vi "Schedule.EditFunction.vi"(8 "error in (no error)":errorcluster, 10 "Settings":string, 11 "ObjectSettings in":refnum<class "ObjectSettings.lvclass">) -> (0 "error out":errorcluster, 2 "Settings Out":string, 3 "ObjectSettings out":refnum<class "ObjectSettings.lvclass">)   [LabVIEW 2019, in "ObjectSettings.lvclass"]
uses:
  ObjectSettings.lvclass
  <vilib>/measure/NI_MABase.lvlib
  subVIs/typedefs/Schedule Types/Schedule--Function Generator.ctl
panel:
  out "Waveform Graph":dbl[](graph)
  in  "Signal Type":T1(ring) caption="Enum"
  in  "Duty Cycle (%)":dbl caption="Numeric"
  in  "Cycle Number":dbl caption="Numeric"
  in  "Max":dbl caption="Numeric"
  in  "Samples (Testing)":dbl caption="Numeric"
  in  "Min":dbl caption="Numeric"
  in  "Phase":dbl caption="Numeric"
  in  "Frequency":dbl caption="Numeric"
  in  "OK":bool
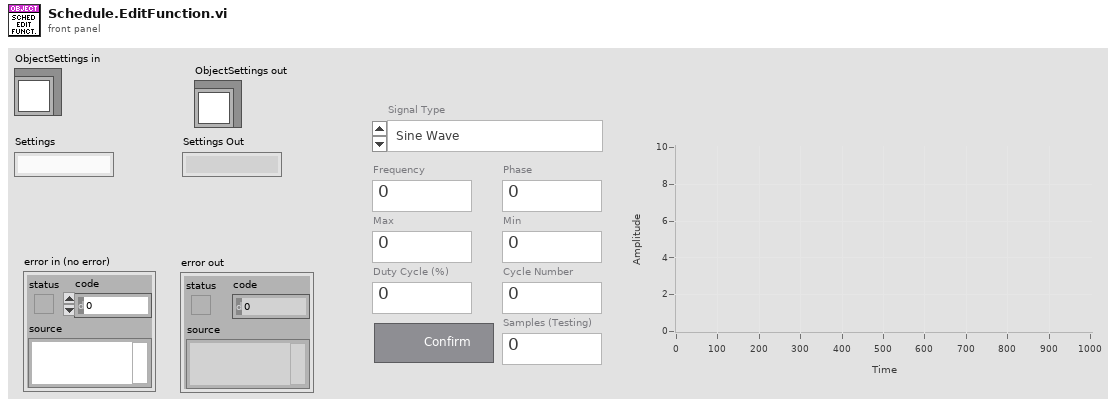
[diagram p1: front panel]
types:
  T1 = enum16{"Sine Wave", "Triangle Wave", "Square Wave", "Sawtooth Wave"}
  T2 = enum32{"Invalid", "Standard", "Closed", "Hidden", "Minimized", "Maximized"}
  T3 = enum32{"invalid app kind", "Development System", "Run Time System", "Student Edition", "Embedded LabVIEW", "Evaluation", "Custom"}
  T4 = typedef "Schedule--Function Generator.ctl" = cluster{"Min Value":dbl, "Max Value":dbl, "Duty Cycle (%)":dbl, "Signal Type":u16, "Cycle Number":dbl, "Phase (degrees)":dbl}
  T5 = cluster{"Core":cluster{"Current VI Reference":refnum<vi>, "Close Panel on Exit?":bool}, "ObjectSettings":refnum<class "ObjectSettings.lvclass">, "Settings":string, "Signal Type":enum16{"Sine Wave", "Triangle Wave", "Square Wave", "Sawtooth Wave"}, "Frequency":dbl, "Max":dbl, "Min":dbl, "Phase":dbl, "Samples (Testing)":dbl, "Cycle Number":dbl, "Duty Cycle (%)":dbl}
  T6 = cluster{"Current VI Reference":refnum<vi>, "Close Panel on Exit?":bool}
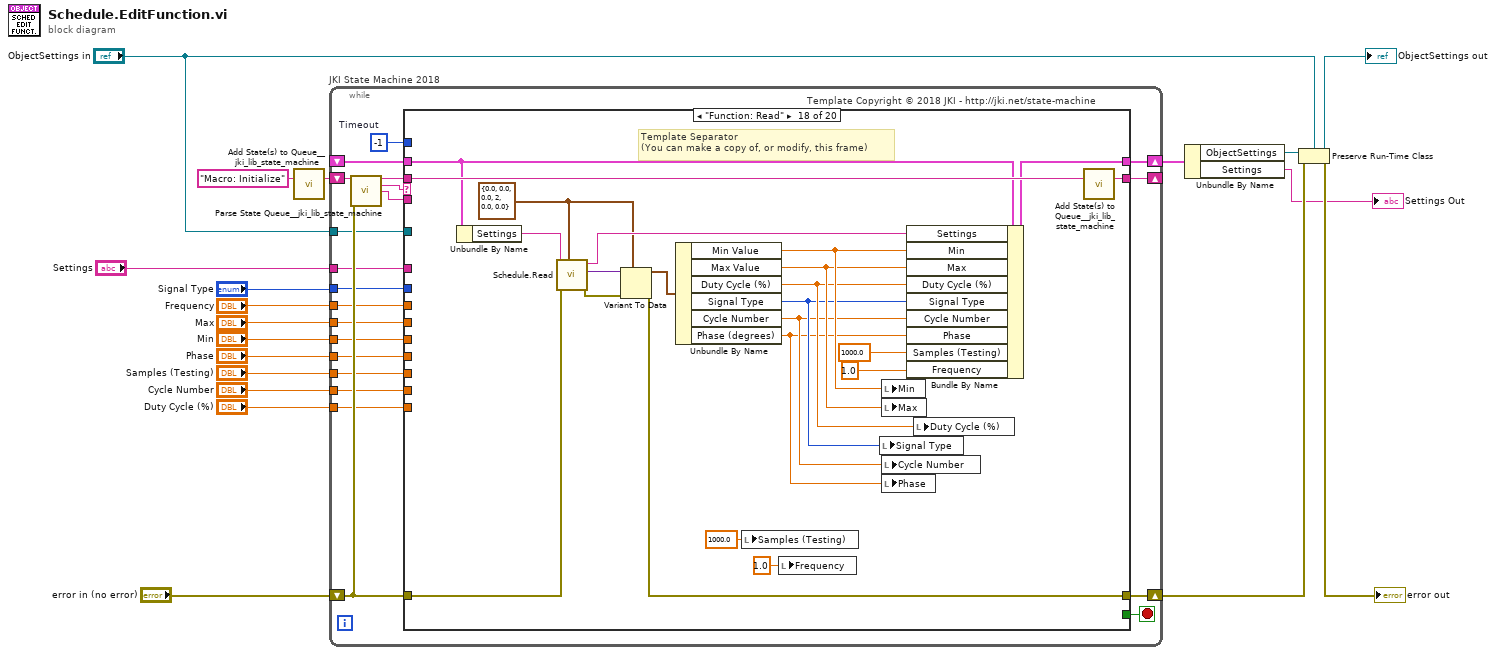
[diagram p0: block diagram]
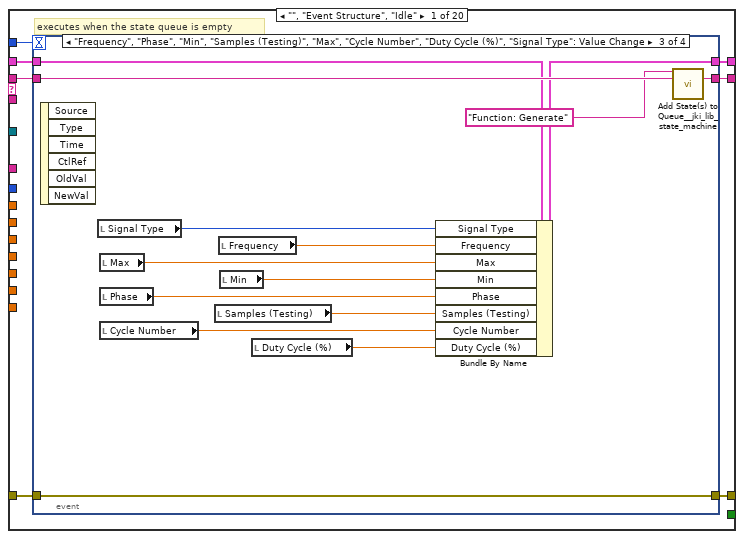
[diagram p2: hidden frame]
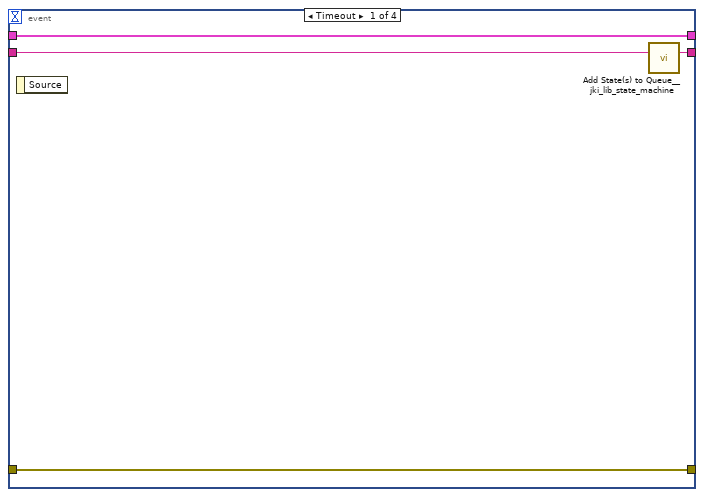
[diagram p3: hidden frame]
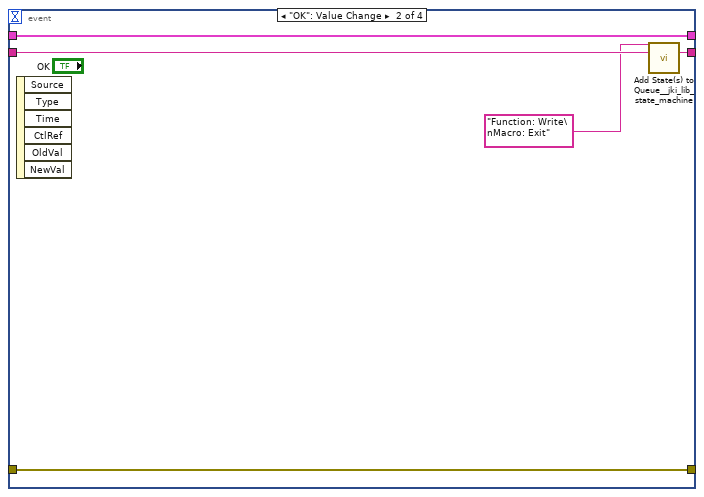
[diagram p4: hidden frame]
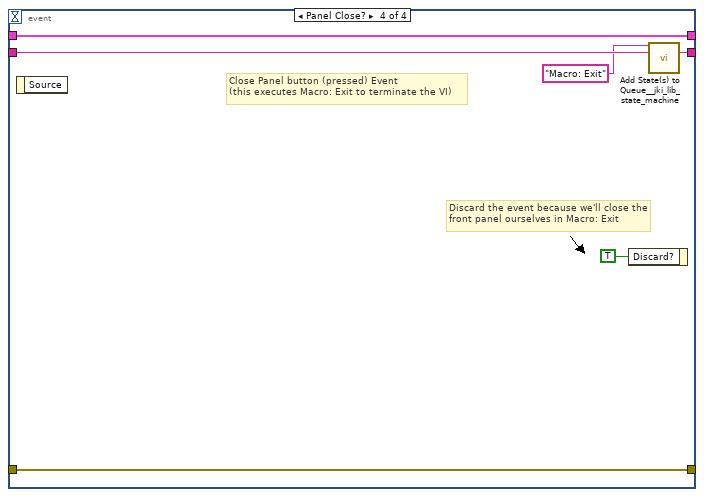
[diagram p5: hidden frame]
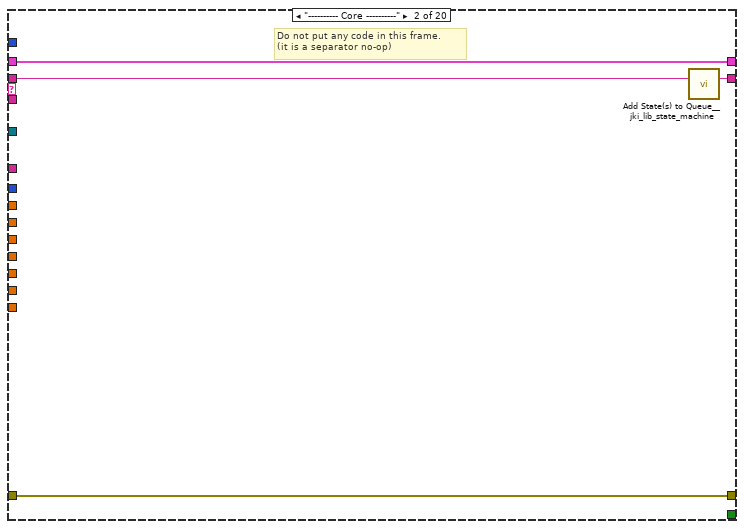
[diagram p6: hidden frame]
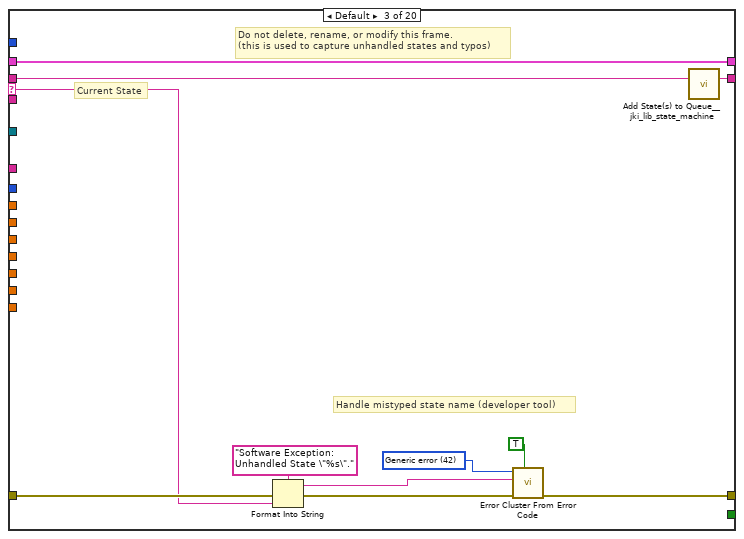
[diagram p7: hidden frame]
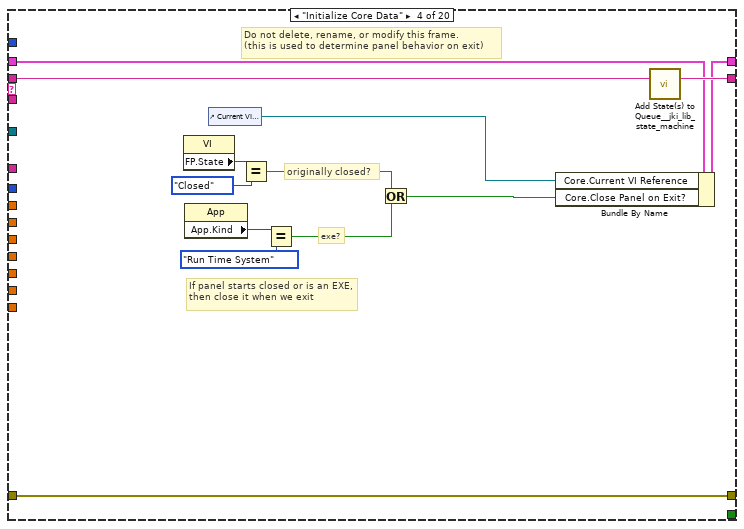
[diagram p8: hidden frame]
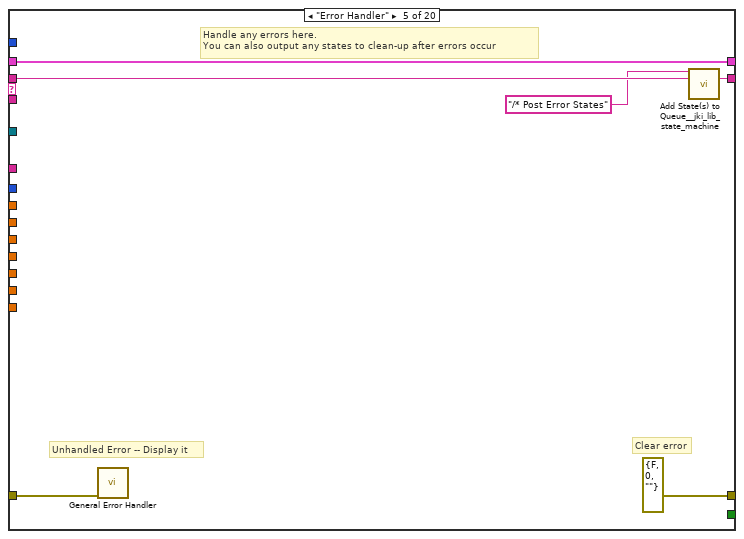
[diagram p9: hidden frame]
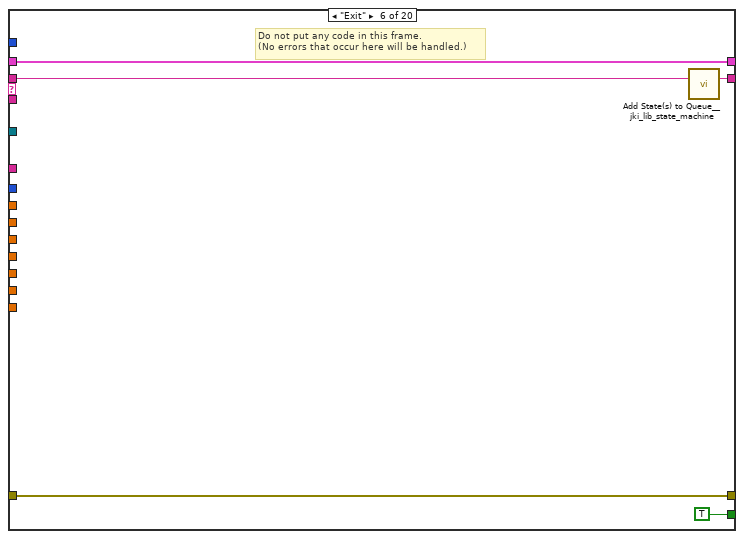
[diagram p10: hidden frame]
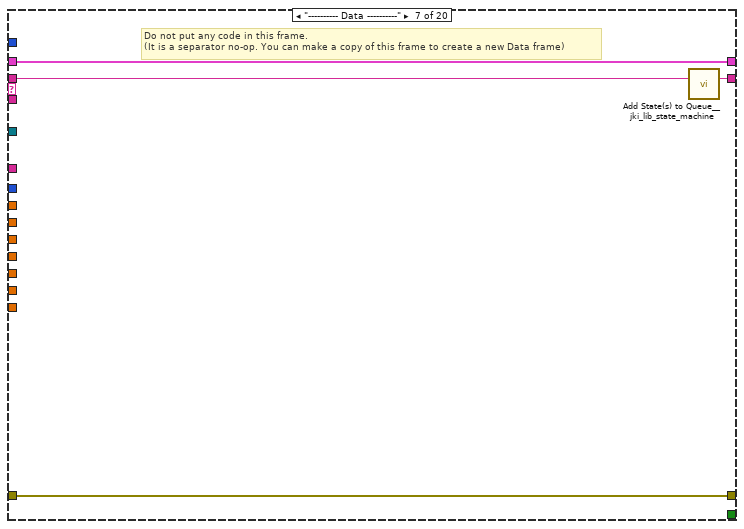
[diagram p11: hidden frame]
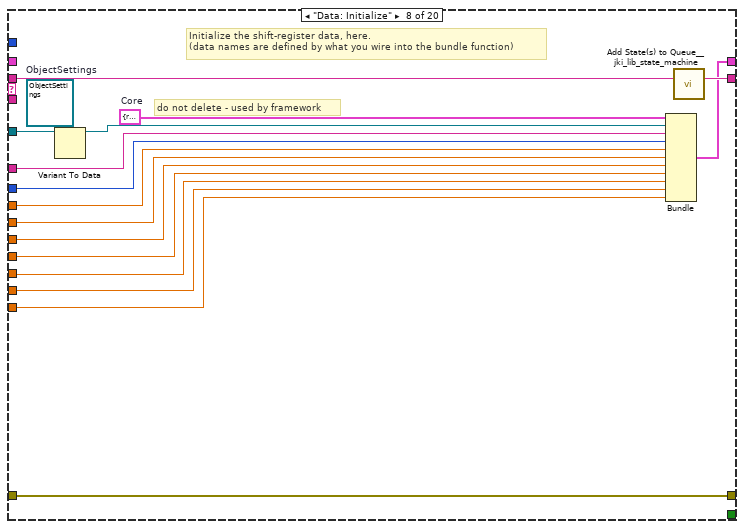
[diagram p12: hidden frame]
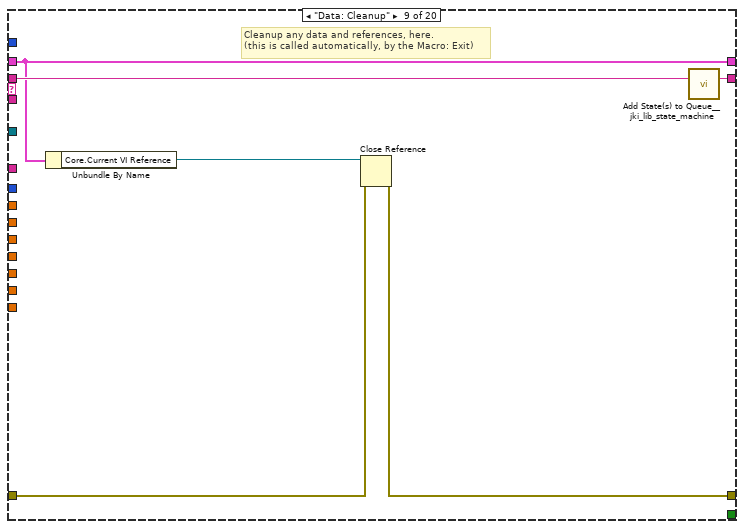
[diagram p13: hidden frame]
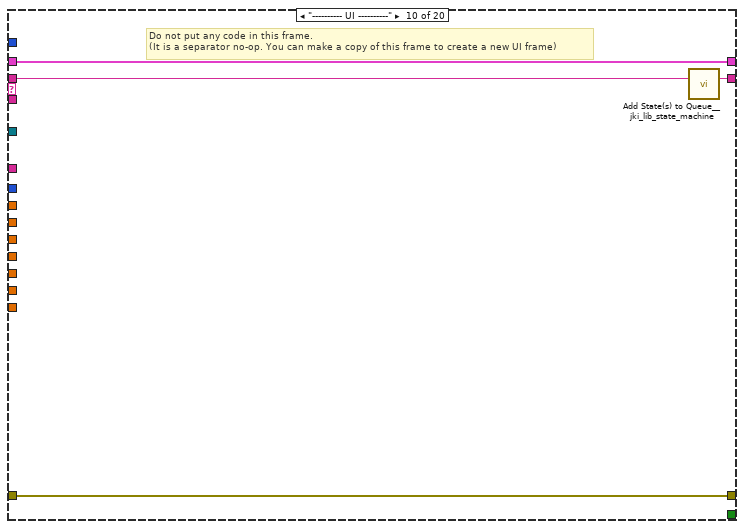
[diagram p14: hidden frame]
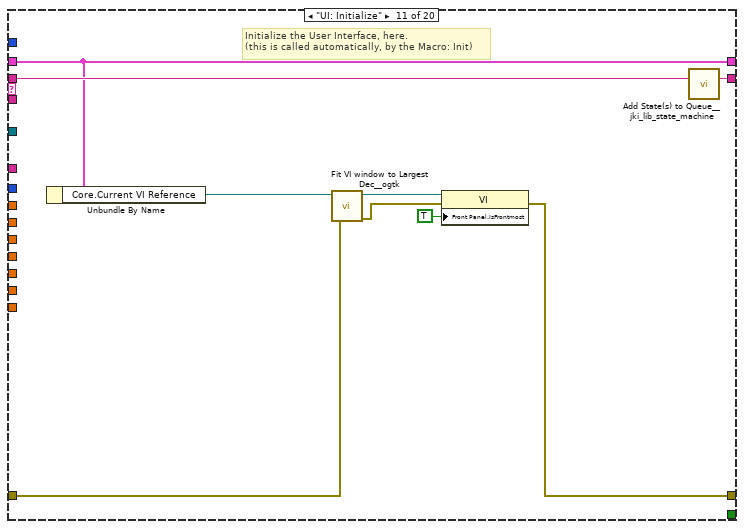
[diagram p15: hidden frame]
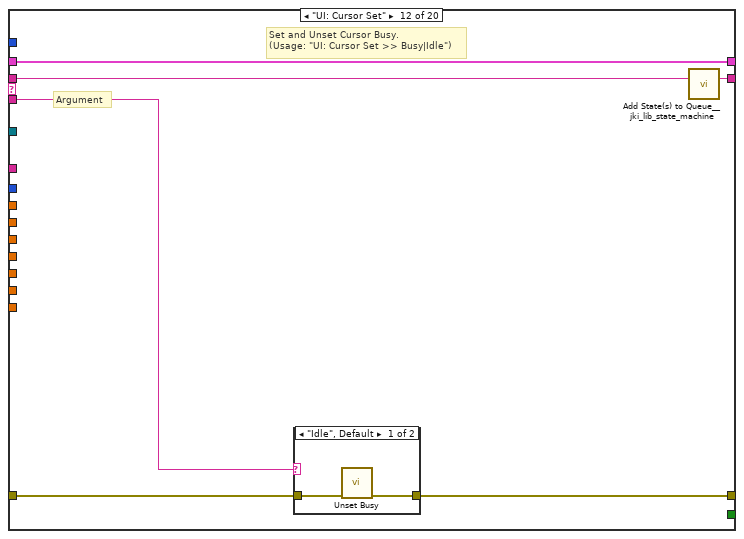
[diagram p16: hidden frame]
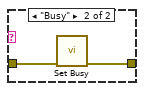
[diagram p17: hidden frame]
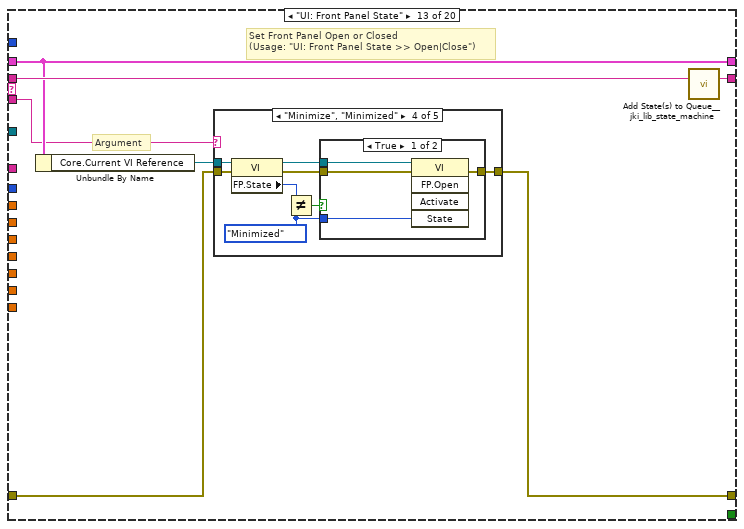
[diagram p18: hidden frame]
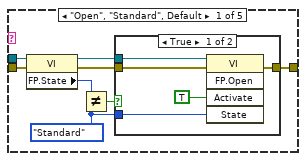
[diagram p19: hidden frame]
diagram:
  n1 = call <vilib>:"Add State(s) to Queue__jki_lib_state_machine.vi"("State(s) in (\"\")"="Macro: Initialize") -> ("States Out"=w19:string)  [unwired: 14 in]
  n2 = while "JKI State Machine 2018" {
    shift-right: [w33] -> w15
    shift-left: _ -> [w32]
    shift-right: [w36] -> w12
    shift-left: "error in (no error)" -> [w30]
    shift-right: [w35] -> _
    shift-left: w19 -> [w37]
    tunnel: "ObjectSettings in" -> [w29]
    tunnel: "Settings" -> [w28]
    tunnel: "Signal Type" -> [w27]
    tunnel: "Frequency" -> [w26]
    tunnel: "Max" -> [w25]
    tunnel: "Min" -> [w24]
    tunnel: "Phase" -> [w23]
    tunnel: "Samples (Testing)" -> [w22]
    tunnel: "Cycle Number" -> [w21]
    tunnel: "Duty Cycle (%)" -> [w20]
    stop <- w34 stop-if-true
    w31 = -1  # Timeout
    # "Template Copyright © 2018 JKI - http://jki.net/state-machine"
    n3 = call <vilib>:"Parse State Queue__jki_lib_state_machine.vi"("State Queue"=w37, "Error In (no error)"=w30) -> ("Remaining States"=w39:string, "Current State"=w40:string, "Arguments"=w38:string)  [unwired: 11 in]
    n4 = case shown="\"Function: Read\"" w40 {
      selector: w40 -> [_ _ w81 _ _ _ _ _ _ _ _ _ _ _ _ _ _ _ _ _]
      tunnel: w39 -> [w47 w80 w85 w104 w110 w115 w119 w136 w142 w146 w155 w161 w172 w241 w246 w256 w260 w282 w298 w321]
      tunnel: w38 -> [_ _ _ _ _ _ _ _ _ _ _ w156 w166 _ _ _ _ _ _ _]
      tunnel: w32 -> [w45 w77 w83 w97 w107 w113 w116 _ w137 w143 w153 w159 w168 w238 w243 w253 w257 w277 w295 w302]
      tunnel: [w44 w78 w87 w101 errorcluster {"status"=FALSE, "code"=0, "source"=""} ("error out") w112 w117 w133 w138 w144 w147 w157 w169 w239 w244 w254 w258 w263 w283 w319] -> w36
      tunnel: w30 -> [w43 w78 w86 w101 w106 w112 w117 w133 w139 w144 w151 w158 w170 w239 w244 w254 w258 w262 w284 w319]
      tunnel: [w46 w79 w84 w103 w109 w114 w118 w135 w141 w145 w154 w160 w171 w240 w245 w255 w259 w281 w297 w320] -> w35
      tunnel: [_ _ _ _ _ TRUE _ _ _ _ _ _ _ _ _ _ _ _ _ _] -> w34
      tunnel: [w42 w77 w83 w102 w107 w113 w116 w134 w137 w143 w153 w159 w168 w238 w243 w253 w257 w278 w296 w302] -> w33
      tunnel: w31 -> [w41 _ _ _ _ _ _ _ _ _ _ _ _ _ _ _ _ _ _ _]
      tunnel: w29 -> [_ _ _ _ _ _ _ w129 _ _ _ _ _ _ _ _ _ _ _ _]
      tunnel: w28 -> [_ _ _ _ _ _ _ w128 _ _ _ _ _ _ _ _ _ _ _ _]
      tunnel: w27 -> [_ _ _ _ _ _ _ w127 _ _ _ _ _ _ _ _ _ _ _ _]
      tunnel: w26 -> [_ _ _ _ _ _ _ w126 _ _ _ _ _ _ _ _ _ _ _ _]
      tunnel: w25 -> [_ _ _ _ _ _ _ w125 _ _ _ _ _ _ _ _ _ _ _ _]
      tunnel: w24 -> [_ _ _ _ _ _ _ w124 _ _ _ _ _ _ _ _ _ _ _ _]
      tunnel: w23 -> [_ _ _ _ _ _ _ w123 _ _ _ _ _ _ _ _ _ _ _ _]
      tunnel: w22 -> [_ _ _ _ _ _ _ w122 _ _ _ _ _ _ _ _ _ _ _ _]
      tunnel: w21 -> [_ _ _ _ _ _ _ w121 _ _ _ _ _ _ _ _ _ _ _ _]
      tunnel: w20 -> [_ _ _ _ _ _ _ w120 _ _ _ _ _ _ _ _ _ _ _ _]
      frame "", "Event Structure", "Idle" {
        # "executes when the state queue is empty"
        n5 = event shown="[2] \"Frequency\", \"Phase\", \"Min\", \"Samples (Testing)\", \"Max\", \"Cycle Number\", \"Duty Cycle (%)\", \"Signal Type\": Value Change" {
          selector: _ -> [_ _ _ _]
          dyn-events: _ -> [_ _ _ _]
          timeout: w41 -> [_ _ _ _]
          tunnel: w47 -> [w51 w56 w70 w76]
          tunnel: [w50 w55 w69 w75] -> w46
          tunnel: w45 -> [w48 w53 w66 w73]
          tunnel: [w49 w54 w68 w74] -> w44
          tunnel: w43 -> [w49 w54 w68 w74]
          tunnel: [w48 w53 w67 w73] -> w42
          event Timeout {
            n6 = event-data() -> ()  [unwired: 1 in, 1 out]
            n7 = call <vilib>:"Add State(s) to Queue__jki_lib_state_machine.vi"("State(s) in (\"\")"=w51) -> ("States Out"=w50:string)  [unwired: 14 in]
          }
          event "OK": Value Change {
            n8 = event-data() -> ()  [unwired: 1 in, 6 out]
            n9 = call <vilib>:"Add State(s) to Queue__jki_lib_state_machine.vi"("State(s) in Front (\"\")"="Function: Write\nMacro: Exit", "State(s) in (\"\")"=w56) -> ("States Out"=w55:string)  [unwired: 13 in]
          }
          event "Frequency", "Phase", "Min", "Samples (Testing)", "Max", "Cycle Number", "Duty Cycle (%)", "Signal Type": Value Change {
            n10 = event-data() -> ()  [unwired: 1 in, 6 out]
            n11 = local read "Signal Type"() -> (w65:T1)
            n12 = local read "Max"() -> (w63:dbl)
            n13 = local read "Phase"() -> (w58:dbl)
            n14 = local read "Cycle Number"() -> (w60:dbl)
            n15 = local read "Samples (Testing)"() -> (w59:dbl)
            n16 = local read "Frequency"() -> (w64:dbl)
            n17 = local read "Min"() -> (w62:dbl)
            n18 = local read "Duty Cycle (%)"() -> (w61:dbl)
            n19 = Bundle By Name(cluster=w66, "Signal Type"=w65, "Frequency"=w64, "Max"=w63, "Min"=w62, "Phase"=w58, "Samples (Testing)"=w59, "Cycle Number"=w60, "Duty Cycle (%)"=w61) -> (w67:T5)
            n20 = call <vilib>:"Add State(s) to Queue__jki_lib_state_machine.vi"("State(s) in Front (\"\")"="Function: Generate", "State(s) in (\"\")"=w70) -> ("States Out"=w69:string)  [unwired: 13 in]
          }
          event Panel Close? {
            # "Discard the event because we'll close the front panel ourselves in Macro: Exit"
            # "Close Panel button (pressed) Event\n(this executes Macro: Exit to terminate the VI)"
            n21 = event-data() -> ()  [unwired: 1 in, 1 out]
            n22 = event-data("Discard?"=TRUE) -> ()  [unwired: 1 in, 1 out]
            n23 = call <vilib>:"Add State(s) to Queue__jki_lib_state_machine.vi"("State(s) in Front (\"\")"="Macro: Exit", "State(s) in (\"\")"=w76) -> ("States Out"=w75:string)  [unwired: 13 in]
          }
        }
      }
      frame "---------- Core ----------" {
        # "Do not put any code in this frame.\n(it is a separator no-op)"
        n24 = call <vilib>:"Add State(s) to Queue__jki_lib_state_machine.vi"("State(s) in (\"\")"=w80) -> ("States Out"=w79:string)  [unwired: 14 in]
      }
      frame Default {
        w90 = 42 items=["No error", "Argument error", "Memory is full", "Out of zone", "End of file", "File already open", "Generic file I/O error", "File not found", "File permission error", "Disk is full", "Duplicate path", "Too many files open", "System feature not enabled", "Resource file not found", "Cannot add resource", "Resource not found", "Image not found", "Image memory error", "Pen does not exist", "Config type invalid", "Config token not found", "Config parse error", "Config memory error", "Bad external code format", "Bad external code offset", "External code not present", "Null window", "Destroy window error", "Null menu", "Print aborted", "Bad print record", "Print driver error", "Windows error during printing", "Memory error during printing", "Print dialog error", "Generic print error", "Invalid device refnum", "Device not found", "Device parameter error", "Device unit error", "Cannot open device", "Device call aborted", "Generic error", "Cancelled by user", "Object ID too low", "Object ID too high", "Object not in heap", "Unknown heap", "Unknown object (invalid DefProc)", "Unknown object (DefProc not in table)", "Message out of range", "Invalid (null) method", "Unknown message", "Manager call not supported", "Bad address", "Network operation in progress", "Network operation timed out", "Connection is busy", "Network attribute not supported", "Network error", "Address in use", "System out of memory", "Connection aborted", "Connection refused", "Not connected", "Already connected", "Connection closed", "Initialization error (interapplication manager)", "Bad occurrence", "Wait on unbound occurrence handler", "Occurrence queue overflow", "Datalog type conflict", "Unused", "Unrecognized type (interapplication manager)", "Memory corrupt", "Failed to make temporary DLL", "Old CIN version", "Drag socket not found", "Failed to load drop-object", "Failed to register OLE object", "Failed to release OLE object", "Format specifier type mismatch", "Unknown format specifier", "Too few format specifiers", "Too many format specifiers", "Scan failed", "Newer CIN version", "Error converting to variant", "Runtime menu error", "Password tampered", "Variant attribute not found", "Incompatible variant data type", "Event data is not available", "Event Store is not present", "Occurrence is not found", "Event Queue is not created", "Event info is not available", "Refnum passed is NULL", "Error retrieving Class GUID", "Error retrieving CoClass GUID", "Error retrieving TypeLib GUID.", "Bad built application magic bytes.", "Specific driver is different from the specific driver associated with the Logical Name.", "There is no session opened to the class driver.", "Max Error", "MAX - Error with config objects", "MAX - Error loading configuration", "MAX - Group not supported"]
        # "Current State"
        # "Do not delete, rename, or modify this frame.\n(this is used to capture unhandled states and typos)"
        # "Handle mistyped state name (developer tool)"
        n25 = Format Into String(format string="Software Exception: Unhandled State \"%s\"." ("message"), error in=w86, w81) -> (resulting string=w89:string, error out=w88:errorcluster)  [unwired: 1 in]
        n26 = call <vilib>:"Error Cluster From Error Code.vi"("show call chain? (False)"=TRUE, "error in (no error)"=w88, "error message (\"\")"=w89, "error code (0)"=w90) -> ("error out"=w87:errorcluster)  [unwired: 5 in]
        n27 = call <vilib>:"Add State(s) to Queue__jki_lib_state_machine.vi"("State(s) in (\"\")"=w85) -> ("States Out"=w84:string)  [unwired: 14 in]
      }
      frame "Initialize Core Data" {
        # "Do not delete, rename, or modify this frame.\n(this is used to determine panel behavior on exit)"
        # "originally closed?"
        # "exe?"
        # "If panel starts closed or is an EXE, then close it when we exit"
        n28 = property class="VI"() -> ("FP.State"=w94:T2)  [unwired: 2 in, 2 out]
        n29 = property class="App"() -> ("App.Kind"=w100:T3)  [unwired: 2 in, 2 out]
        n30 = control-ref of="Current VI Reference"() -> (w95:refnum<vi>)
        n31 = Equal?(x=w94, y=T2."Closed" ("Front Panel Window:State")) -> (x = y?=w92:bool)
        n32 = Equal?(x=w100, y=T3."Run Time System" ("Application:Kind")) -> (x = y?=w98:bool)
        n33 = Or(x=w92, y=w98) -> (x .or. y?=w96:bool)
        n34 = Bundle By Name(cluster=w97, "Core.Current VI Reference"=w95, "Core.Close Panel on Exit?"=w96) -> (w102:T5)
        n35 = call <vilib>:"Add State(s) to Queue__jki_lib_state_machine.vi"("State(s) in (\"\")"=w104) -> ("States Out"=w103:string)  [unwired: 14 in]
      }
      frame "Error Handler" {
        # "Unhandled Error -- Display it"
        # "Handle any errors here.\nYou can also output any states to clean-up after errors occur"
        # "Clear error"
        n36 = call <vilib>:"General Error Handler.vi"("error in (no error)"=w106) -> ()  [unwired: 10 in, 5 out]
        n37 = call <vilib>:"Add State(s) to Queue__jki_lib_state_machine.vi"("State(s) in Front (\"\")"="/* Post Error States", "State(s) in (\"\")"=w110) -> ("States Out"=w109:string)  [unwired: 13 in]
      }
      frame "Exit" {
        # "Do not put any code in this frame.\n(No errors that occur here will be handled.)"
        n38 = call <vilib>:"Add State(s) to Queue__jki_lib_state_machine.vi"("State(s) in (\"\")"=w115) -> ("States Out"=w114:string)  [unwired: 14 in]
      }
      frame "---------- Data ----------" {
        # "Do not put any code in this frame.\n(It is a separator no-op. You can make a copy of this frame to create a new Data frame)"
        n39 = call <vilib>:"Add State(s) to Queue__jki_lib_state_machine.vi"("State(s) in (\"\")"=w119) -> ("States Out"=w118:string)  [unwired: 14 in]
      }
      frame "Data: Initialize" {
        w130 = refnum<class "ObjectSettings.lvclass"> refnum  # ObjectSettings
        w132 = T6 {"Current VI Reference"=refnum, "Close Panel on Exit?"=TRUE}  # Core
        # "do not delete - used by framework"
        # "Initialize the shift-register data, here.\n(data names are defined by what you wire into the bundle function)"
        n40 = Variant To Data(type=w130, Variant=w129) -> (data=w131:refnum<class "ObjectSettings.lvclass">)  [unwired: 1 in, 1 out]
        n41 = Bundle("Core"=w132, "ObjectSettings"=w131, "Settings"=w128, "Signal Type"=w127, "Frequency"=w126, "Max"=w125, "Min"=w124, "Phase"=w123, "Samples (Testing)"=w122, "Cycle Number"=w121, "Duty Cycle (%)"=w120) -> (w134:T5)  [unwired: 1 in]
        n42 = call <vilib>:"Add State(s) to Queue__jki_lib_state_machine.vi"("State(s) in (\"\")"=w136) -> ("States Out"=w135:string)  [unwired: 14 in]
      }
      frame "Data: Cleanup" {
        # "Cleanup any data and references, here.\n(this is called automatically, by the Macro: Exit)"
        n43 = Unbundle By Name(w137) -> ("Core.Current VI Reference"=w140:refnum<vi>)
        n44 = Close Reference(reference=w140, error in (no error)=w139) -> (error out=w138:errorcluster)
        n45 = call <vilib>:"Add State(s) to Queue__jki_lib_state_machine.vi"("State(s) in (\"\")"=w142) -> ("States Out"=w141:string)  [unwired: 14 in]
      }
      frame "---------- UI ----------" {
        # "Do not put any code in this frame.\n(It is a separator no-op. You can make a copy of this frame to create a new UI frame)"
        n46 = call <vilib>:"Add State(s) to Queue__jki_lib_state_machine.vi"("State(s) in (\"\")"=w146) -> ("States Out"=w145:string)  [unwired: 14 in]
      }
      frame "UI: Initialize" {
        # "Initialize the User Interface, here.\n(this is called automatically, by the Macro: Init)"
        n47 = Unbundle By Name(w153) -> ("Core.Current VI Reference"=w152:refnum<vi>)
        n48 = call <userlib>:"Fit VI window to Largest Dec__ogtk.vi"("error in (no error)"=w151, "VI Ref (calling VI)"=w152) -> ("error out"=w148:errorcluster, "dup VI Ref"=w149:refnum<vi>)  [unwired: 4 in]
        n49 = property class="VI"(reference=w149, error in=w148, "Front Panel.IsFrontmost"=TRUE ("Front Panel Window:Is Frontmost")) -> (error out=w147:errorcluster)  [unwired: 1 out]
        n50 = call <vilib>:"Add State(s) to Queue__jki_lib_state_machine.vi"("State(s) in (\"\")"=w155) -> ("States Out"=w154:string)  [unwired: 14 in]
      }
      frame "UI: Cursor Set" {
        # "Argument"
        # "Set and Unset Cursor Busy.\n(Usage: \"UI: Cursor Set >> Busy|Idle\")"
        n51 = case shown="\"Idle\", Default" w156 {
          tunnel: w158 -> [w163 w165]
          tunnel: [w162 w164] -> w157
          frame "Idle", Default {
            n52 = call <vilib>:"Unset Busy.vi"("error in (no error)"=w163) -> ("error out"=w162:errorcluster)  [unwired: 10 in]
          }
          frame "Busy" {
            n53 = call <vilib>:"Set Busy.vi"("error in (no error)"=w165) -> ("error out"=w164:errorcluster)  [unwired: 9 in, 1 out]
          }
        }
        n54 = call <vilib>:"Add State(s) to Queue__jki_lib_state_machine.vi"("State(s) in (\"\")"=w161) -> ("States Out"=w160:string)  [unwired: 14 in]
      }
      frame "UI: Front Panel State" {
        # "Argument"
        # "Set Front Panel Open or Closed\n(Usage: \"UI: Front Panel State >> Open|Close\")"
        n55 = Unbundle By Name(w168) -> ("Core.Current VI Reference"=w167:refnum<vi>)
        n56 = case shown="\"Minimize\", \"Minimized\"" w166 {
          tunnel: w170 -> [w178 w193 w204 w217 w230]
          tunnel: [w180 w194 w206 w219 w232] -> w169
          tunnel: w167 -> [w179 w191 w205 w218 w231]
          frame "Open", "Standard", Default {
            w173 = T2."Standard" ("State")
            n57 = property class="VI"(reference=w179, error in=w178) -> (reference out=w176:refnum<vi>, error out=w177:errorcluster, "FP.State"=w175:T2)
            n58 = Not Equal?(x=w175, y=w173) -> (x != y?=w174:bool)
            n59 = case shown="True" w174 {
              tunnel: [w184 w186] -> w180
              tunnel: w177 -> [w183 w186]
              tunnel: w176 -> [w182 _]
              tunnel: w173 -> [w181 _]
              frame True {
                n60 = invoke class="VI" method="FP.Open"(reference=w182, error in=w183, "Activate"=TRUE, "State"=w181) -> (error out=w184:errorcluster)  [unwired: 1 in, 4 out]
              }
              frame False {
              }
            }
          }
          frame "Close", "Closed" {
            n61 = property class="VI"(reference=w191, error in=w193) -> (reference out=w190:refnum<vi>, error out=w192:errorcluster, "FP.State"=w188:T2)
            n62 = Not Equal?(x=w188, y=T2."Closed" ("Front Panel Window:State")) -> (x != y?=w187:bool)
            n63 = case shown="True" w187 {
              tunnel: [w195 w198] -> w194
              tunnel: w192 -> [w195 w197]
              tunnel: w190 -> [_ w196]
              frame False {
              }
              frame True {
                n64 = invoke class="VI" method="FP.Close"(reference=w196, error in=w197) -> (error out=w198:errorcluster)  [unwired: 1 in, 2 out]
              }
            }
          }
          frame "Hidden", "Hide" {
            w199 = T2."Hidden" ("State")
            n65 = property class="VI"(reference=w205, error in=w204) -> (reference out=w202:refnum<vi>, error out=w203:errorcluster, "FP.State"=w201:T2)
            n66 = Not Equal?(x=w201, y=w199) -> (x != y?=w200:bool)
            n67 = case shown="True" w200 {
              tunnel: [w210 w211] -> w206
              tunnel: w203 -> [w209 w211]
              tunnel: w202 -> [w208 _]
              tunnel: w199 -> [w207 _]
              frame True {
                n68 = invoke class="VI" method="FP.Open"(reference=w208, error in=w209, "State"=w207) -> (error out=w210:errorcluster)  [unwired: 2 in, 4 out]
              }
              frame False {
              }
            }
          }
          frame "Minimize", "Minimized" {
            w212 = T2."Minimized" ("State")
            n69 = property class="VI"(reference=w218, error in=w217) -> (reference out=w215:refnum<vi>, error out=w216:errorcluster, "FP.State"=w214:T2)
            n70 = Not Equal?(x=w214, y=w212) -> (x != y?=w213:bool)
            n71 = case shown="True" w213 {
              tunnel: [w223 w224] -> w219
              tunnel: w216 -> [w222 w224]
              tunnel: w215 -> [w221 _]
              tunnel: w212 -> [w220 _]
              frame True {
                n72 = invoke class="VI" method="FP.Open"(reference=w221, error in=w222, "State"=w220) -> (error out=w223:errorcluster)  [unwired: 2 in, 4 out]
              }
              frame False {
              }
            }
          }
          frame "Maximize", "Maximized" {
            w225 = T2."Maximized" ("State")
            n73 = property class="VI"(reference=w231, error in=w230) -> (reference out=w228:refnum<vi>, error out=w229:errorcluster, "FP.State"=w227:T2)
            n74 = Not Equal?(x=w227, y=w225) -> (x != y?=w226:bool)
            n75 = case shown="True" w226 {
              tunnel: [w236 w237] -> w232
              tunnel: w229 -> [w235 w237]
              tunnel: w228 -> [w234 _]
              tunnel: w225 -> [w233 _]
              frame True {
                n76 = invoke class="VI" method="FP.Open"(reference=w234, error in=w235, "State"=w233) -> (error out=w236:errorcluster)  [unwired: 2 in, 4 out]
              }
              frame False {
              }
            }
          }
        }
        n77 = call <vilib>:"Add State(s) to Queue__jki_lib_state_machine.vi"("State(s) in (\"\")"=w172) -> ("States Out"=w171:string)  [unwired: 14 in]
      }
      frame "---------- Macro ----------" {
        # "Do not put any code in this frame.\n(It is a separator no-op. You can make a copy of this frame to create a new Macro frame)"
        n78 = call <vilib>:"Add State(s) to Queue__jki_lib_state_machine.vi"("State(s) in (\"\")"=w241) -> ("States Out"=w240:string)  [unwired: 14 in]
      }
      frame "Macro: Initialize" {
        w242 = "Data: Initialize\nInitialize Core Data\nFunction: Read\nUI: Initialize\nUI: Front Panel State >> Open"  # Data: Initialize Initialize Core Data Function: Read UI: Initialize UI: Front Panel State >> Open
        # "Initialization Macro\n(This is called once, when the VI starts)"
        n79 = call <vilib>:"Add State(s) to Queue__jki_lib_state_machine.vi"("State(s) in Front (\"\")"=w242, "State(s) in (\"\")"=w246) -> ("States Out"=w245:string)  [unwired: 13 in]
      }
      frame "Macro: Exit" {
        # "Exit Macro\n(This is called once, when the VI exits)"
        n80 = Unbundle By Name(w253) -> ("Core.Close Panel on Exit?"=w252:bool)
        n81 = Select(t="UI: Front Panel State >> Close", s=w252, f="") -> (s? t:f=w249:string)
        n82 = call <vilib>:"Add State(s) to Queue__jki_lib_state_machine.vi"("State(s) in (\"\")"=w249, "State(s) at Back (\"\")"="Data: Cleanup\nExit") -> ("States Out"=w247:string)  [unwired: 13 in]
        n83 = call <vilib>:"Add State(s) to Queue__jki_lib_state_machine.vi"("State(s) in Front (\"\")"=w247, "State(s) in (\"\")"=w256) -> ("States Out"=w255:string)  [unwired: 13 in]
      }
      frame "---------- Function ----------" {
        # "Template Separator\n(You can make a copy of, or modify, this frame)"
        n84 = call <vilib>:"Add State(s) to Queue__jki_lib_state_machine.vi"("State(s) in (\"\")"=w260) -> ("States Out"=w259:string)  [unwired: 14 in]
      }
      frame "Function: Read" {
        w265 = T4 {"Min Value"=0.0, "Max Value"=0.0, "Duty Cycle (%)"=0.0, "Signal Type"=2, "Cycle Number"=0.0, "Phase (degrees)"=0.0} ("Fn. Gen")
        # "Template Separator\n(You can make a copy of, or modify, this frame)"
        n85 = Unbundle By Name(w277) -> ("Settings"=w268:string)
        n86 = call "Schedule.Read.vi"("Data to Read"=w265, "error in (no error)"=w262, "Schedule <JSON> In"=w268) -> ("error out"=w261:errorcluster, "Data Out"=w266:variant, "Schedule <JSON> Out"=w267:string)  [unwired: 6 in]
        n87 = Variant To Data(error in=w261, type=w265, Variant=w266) -> (data=w264:T4, error out=w263:errorcluster)
        n88 = Unbundle By Name(w264) -> ("Min Value"=w276:dbl, "Max Value"=w275:dbl, "Duty Cycle (%)"=w274:dbl, "Signal Type"=w273:u16, "Cycle Number"=w272:dbl, "Phase (degrees)"=w271:dbl)
        n89 = local write "Samples (Testing)"(1000.0 ("Samples Testing")) -> ()
        n90 = local write "Frequency"(1.0 ("frequency")) -> ()
        n91 = local write "Signal Type"(w273) -> ()
        n92 = local write "Min"(w276) -> ()
        n93 = local write "Max"(w275) -> ()
        n94 = local write "Cycle Number"(w272) -> ()
        n95 = local write "Phase"(w271) -> ()
        n96 = Bundle By Name(cluster=w277, "Settings"=w267, "Min"=w276, "Max"=w275, "Duty Cycle (%)"=w274, "Signal Type"=w273, "Cycle Number"=w272, "Phase"=w271, "Samples (Testing)"=1000.0 ("Samples Testing"), "Frequency"=1.0 ("frequency")) -> (w278:T5)
        n97 = local write "Duty Cycle (%)"(w274) -> ()
        n98 = call <vilib>:"Add State(s) to Queue__jki_lib_state_machine.vi"("State(s) in (\"\")"=w282) -> ("States Out"=w281:string)  [unwired: 14 in]
      }
      frame "Function: Write" {
        # "Template Separator\n(You can make a copy of, or modify, this frame)"
        n99 = Unbundle By Name(w295) -> ("Settings"=w287:string, "Min"=w293:dbl, "Max"=w292:dbl, "Duty Cycle (%)"=w291:dbl, "Signal Type"=w290:T1, "Cycle Number"=w289:dbl, "Phase"=w288:dbl)
        n100 = Bundle By Name(cluster=T4 {"Min Value"=0.0, "Max Value"=0.0, "Duty Cycle (%)"=0.0, "Signal Type"=2, "Cycle Number"=0.0, "Phase (degrees)"=0.0} ("Fn. Gen"), "Min Value"=w293, "Max Value"=w292, "Duty Cycle (%)"=w291, "Signal Type"=w290, "Cycle Number"=w289, "Phase (degrees)"=w288) -> (w285:T4)
        n101 = call "Schedule.Write.vi"("error in (no error)"=w284, "Data to Write"=w285, "Schedule <JSON> In"=w287) -> ("error out"=w283:errorcluster, "Schedule <JSON> Out"=w286:string)  [unwired: 7 in]
        n102 = Bundle By Name(cluster=w295, "Settings"=w286) -> (w296:T5)
        n103 = call <vilib>:"Add State(s) to Queue__jki_lib_state_machine.vi"("State(s) in (\"\")"=w298) -> ("States Out"=w297:string)  [unwired: 14 in]
      }
      frame "Function: Generate" {
        # "#check\nWhy isnt frequency saved in the settings?"
        # "Your code here.\n(You can make a copy of, or modify, this frame)"
        n104 = Unbundle By Name(w302) -> ("Signal Type"=w308:T1, "Frequency"=w307:dbl, "Max"=w301:dbl, "Min"=w306:dbl, "Phase"=w300:dbl, "Samples (Testing)"=w305:dbl, "Cycle Number"=w304:dbl, "Duty Cycle (%)"=w303:dbl)
        n105 = Divide(x=w305, y=w304) -> (x/y=w317:dbl)
        n106 = Add(x=w301, y=w306) -> (x+y=w311:dbl)
        n107 = Subtract(x=w301, y=w306) -> (x-y=w314:dbl)
        n108 = Bundle By Name(cluster=cluster{"Fs":dbl, "#s":dbl} {"Fs"=1000.0, "#s"=1000.0} ("sampling info"), "#s"=w305, "Fs"=w317) -> (w316:cluster{"Fs":dbl, "#s":dbl})
        n109 = Divide(x=w311, y=2.0) -> (x/y=w309:dbl)
        n110 = Divide(x=w314, y=2.0) -> (x/y=w312:dbl)
        n111 = call <vilib>:"Basic Function Generator.vi"("offset"=w309, "square wave duty cycle (%)"=w303, "sampling info"=w316, "signal type"=w308, "phase"=w300, "amplitude"=w312, "frequency"=w307) -> ("signal out"=w315:waveform(dbl))  [unwired: 2 in, 2 out]
        n112 = Unbundle By Name(w315) -> ("Y"=→"Waveform Graph":dbl[])
        n113 = call <vilib>:"Add State(s) to Queue__jki_lib_state_machine.vi"("State(s) in (\"\")"=w321) -> ("States Out"=w320:string)  [unwired: 14 in]
      }
    }
  }
  n114 = Unbundle By Name(w15) -> ("ObjectSettings"=w13:refnum<class "ObjectSettings.lvclass">, "Settings"=→"Settings Out":string)
  n115 = Preserve Run-Time Class(object in=w13, error in=w12, 2:"ObjectSettings in") -> (object out=→"ObjectSettings out":refnum<class "ObjectSettings.lvclass">, error out=→"error out":errorcluster)
